vi "MusicLoader.vi"() -> ()   [LabVIEW 2019, in "Initializers.lvlib"]
uses:
  Initializers.lvlib
  <vilib>/sound2/lvsound2.llb/Sound File Read Open.vi
  <vilib>/sound2/lvsound2.llb/Sound File Read (DBL).vi
panel:
  out "Waveform Graph":i16[](graph)
  out "error out 2":errorcluster
  in  "error out":errorcluster
  in  "Target Path":path=path "C:/Users/FreshBob/Dropbox/VIs/myRIO_GameConsole/Data/Music/menu.music"
  in  "Paths":path=path "C:/Users/FreshBob/Dropbox/VIs/myRIO_GameConsole/Data/8bitCore.wav"
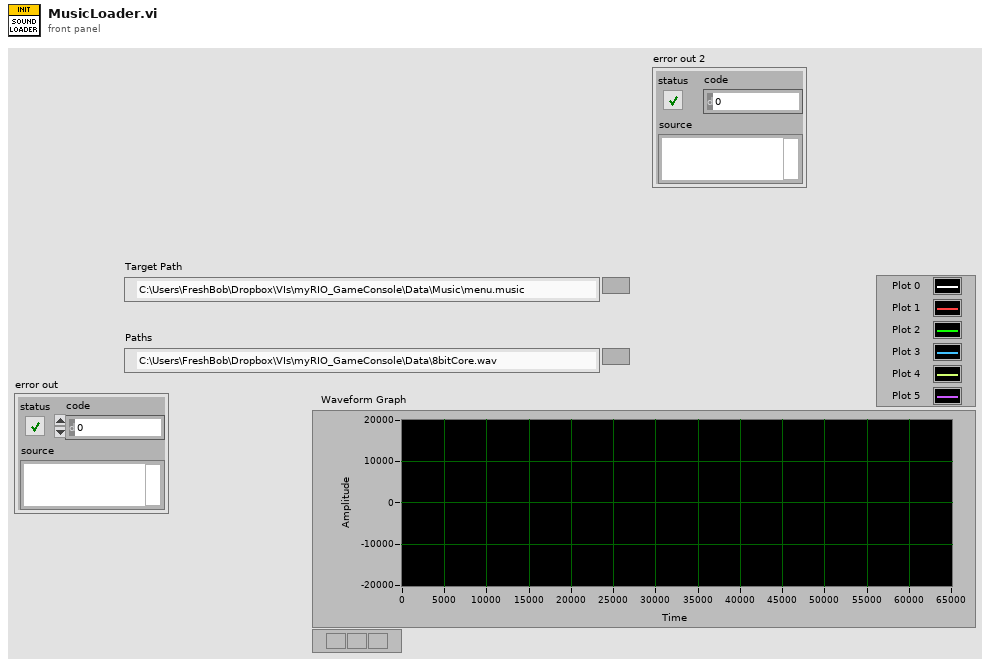
[diagram p1: front panel]
types:
  T1 = enum16{"open", "replace", "create", "open or create", "replace or create", "replace or create with confirmation"}
  T2 = typedef "Sound File Refnum.ctl" = refnum<file>
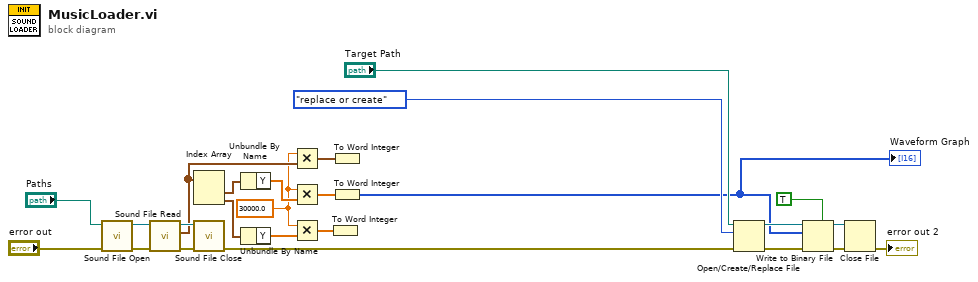
[diagram p0: block diagram]
diagram:
  w2 = 30000.0 ("x")
  n1 = call-poly <vilib>:"Sound File Open.vi"("error in (no error)"="error out", "path"="Paths") -> ("error out"=w13:errorcluster, "sound file refnum"=w14:T2)  [unwired: 8 in]
  n2 = call-poly <vilib>:"Sound File Read.vi"("error in (no error)"=w13, "sound file refnum"=w14) -> ("error out"=w11:errorcluster, "data"=w6:waveform(dbl)[], "sound file refnum out"=w12:T2)  [unwired: 5 in, 2 out]
  n3 = Index Array(array=w6) -> (element #1=w10:waveform(dbl), element #2=w9:waveform(dbl))  [unwired: 2 in]
  n4 = call <vilib>:"Sound File Close.vi"("error in (no error)"=w11, "sound file refnum"=w12) -> ("error out"=w18:errorcluster)  [unwired: 9 in]
  n5 = Unbundle By Name(w10) -> ("Y"=w7:dbl[])
  n6 = Unbundle By Name(w9) -> ("Y"=w8:dbl[])
  n7 = Multiply(x=w2, y=w6) -> (x*y=w3:waveform(dbl)[])
  n8 = Multiply(x=w2, y=w7) -> (x*y=w5:dbl[])
  n9 = Multiply(x=w2, y=w8) -> (x*y=w4:dbl[])
  n10 = To Word Integer(number=w4) -> ()  [unwired: 1 out]
  n11 = To Word Integer(number=w3) -> ()  [unwired: 1 out]
  n12 = To Word Integer(number=w5) -> (16bit integer=w1:i16[])
  "Waveform Graph" <- w1
  n13 = Open/Create/Replace File(file path (use dialog)="Target Path", error in=w18, operation (0:open)=T1."replace or create") -> (refnum out=w25:refnum<file>, error out=w24:errorcluster)  [unwired: 3 in, 1 out]
  n14 = Write to Binary File(file (use dialog)=w25, data=w1, error in=w24, 5:TRUE ("prepend array or string size? (T)")) -> (refnum out=w23:refnum<file>, error out=w22:errorcluster)  [unwired: 2 in, 1 out]
  n15 = Close File(refnum=w23, error in=w22) -> (error out=→"error out 2":errorcluster)  [unwired: 1 out]
